vi "New.vi"(8 "error in (no error)":errorcluster, 11 "reference in":refnum<class "LCR_BK891.lvclass">) -> (0 "error out":errorcluster, 3 "reference out":refnum<class "LCR_BK891.lvclass">)   [LabVIEW 2022 SP3, in "LCR_BK891.lvlib" / "LCR_BK891.lvclass"]
uses:
  LCR_BK891.lvclass
  ObjectAttributes.ctl
  Config.ctl
  LCR_BK891.lvclass/LCR_BK891.ctl
  Components/ViPER.lvlibp/ViPER.lvclass
panel:
  in  "Data":T1={"Config"={"VISA"=""}, "VISA Ref"="", "Function"=4, "Range"=1, "Measurement Speed"=2, "Signal Frequency"=1000.0, "Signal Level"=0, "Measured Primary Reading"=0.0, "Measured Secondary Reading"=0.0} {"Signal Level" items=["0.5Vrms", "1Vrms"]; "Signal Frequency" format="%#_4g"; "Measurement Speed" items=["Slow"=1, "Fast"=2]; "Range" items=["Hold", "Auto"]; "Function" items=["Cs-Q", "Cs-D", "Cs-R", "Cp-Q", "Cp-D", "Cp-R", "Cp-G", "Ls-Q", "Ls-D", "Ls-R", "Lp-Q", "Lp-D", "Lp-R", "Lp-G", "Z-th", "Y-th", "R-X", "G-B", "DCR"]}
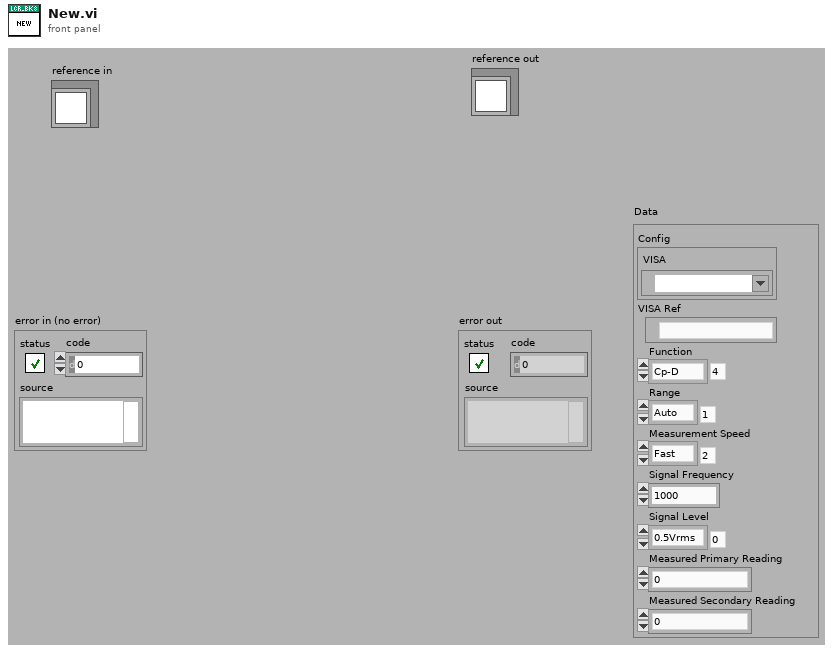
[diagram p1: front panel]
types:
  T1 = typedef "LCR_BK891.lvlib/LCR_BK891.lvclass/ObjectAttributes.ctl" = cluster{"Config":T2, "VISA Ref":refnum<visa-resource-name>, "Function":u16, "Range":u16, "Measurement Speed":u16, "Signal Frequency":dbl, "Signal Level":u8, "Measured Primary Reading":dbl, "Measured Secondary Reading":dbl}
  T2 = typedef "LCR_BK891.lvlib/LCR_BK891.lvclass/Config.ctl" = cluster{"VISA":refnum<visa-resource-name>}
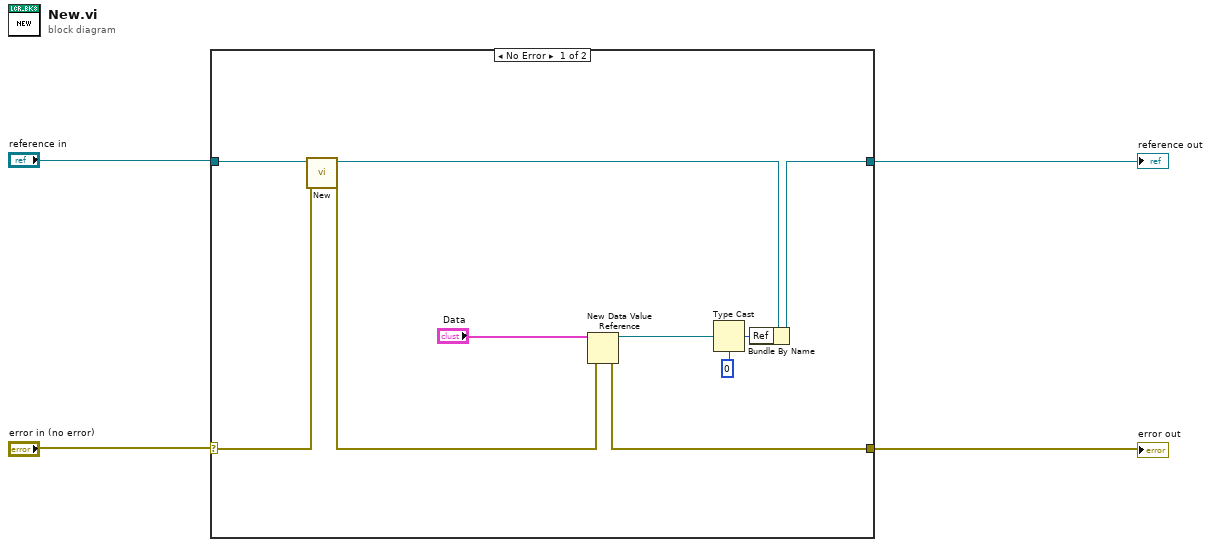
[diagram p0: block diagram]
diagram:
  n1 = case shown="No Error" "error in (no error)" {
    selector: "error in (no error)" -> [w6 w16]
    tunnel: [w7 w16] -> w2
    tunnel: "reference in" -> [w14 w15]
    tunnel: [w13 w15] -> w1
    frame No Error {
      n2 = call-parent "New.vi"("error in (no error)"=w6, "reference in"=w14) -> ("error out"=w5:errorcluster, "reference out"=w12:refnum<class "LCR_BK891.lvclass">)  [unwired: 8 in]
      n3 = New Data Value Reference(data value="Data", error in=w5) -> (data value reference=w10:refnum<data-value>, error out=w7:errorcluster)
      n4 = Type Cast(type=u32 0 ("DataRef"), x=w10) -> (*(type *) &x=w9:u32)
      n5 = Bundle By Name(cluster=w12, "Ref"=w9) -> (w13:refnum<class "LCR_BK891.lvclass">)
    }
    frame Error {
    }
  }
  "error out" <- w2
  "reference out" <- w1
